vi "RTMain.Write Data.vi"(8 "error in":errorcluster, 9 "WriteUpdate":refnum<k33>, 10 "Read from VS Engine FIFO":refnum<k33>, 11 "Data Refs":T1 {"Write Refs" format="%.0x"; "Read Refs" format="%.0x"}) -> (0 "error out":errorcluster, 3 "Data Refs":T1 {"Write Refs" format="%.0x"; "Read Refs" format="%.0x"})   [LabVIEW 2019, in "OPC UA Client Engine.lvlib"]
uses:
  OPC UA Client Engine.lvlib
  Shared/Tags.ReadWriteRefs.ctl
  <vilib>/NI VeriStand/Custom Device API/Data Reference.ctl
  <vilib>/NI VeriStand/Custom Device API/Global Data Refs.vi
  <vilib>/NI VeriStand/Custom Device API/Custom Device API.lvlib
  Shared/OPC UA Client Shared.lvlib
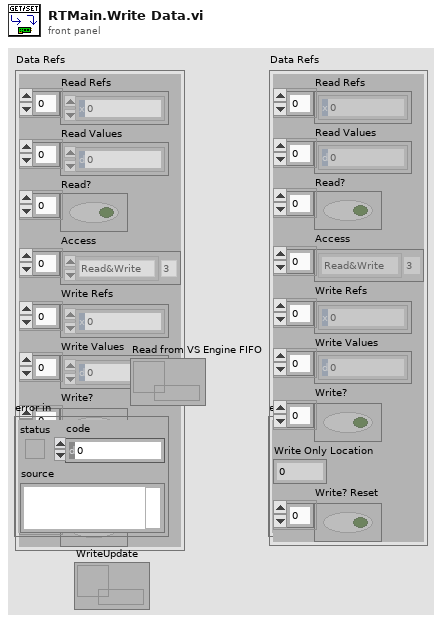
[diagram p1: front panel]
types:
  T1 = typedef "OPC UA Client Shared.lvlib/Tags.ReadWriteRefs.ctl" = cluster{"Read Refs":T2[], "Read Values":dbl[], "Read?":bool[], "Access":enum8{"Null", "Read", "Write", "Read&Write"}[], "Write Refs":T2[], "Write Values":dbl[], "Write?":bool[], "Write Only Location":u32, "Write? Reset":bool[]}
  T2 = typedef "Custom Device API.lvlib/Data Reference.ctl" = i32
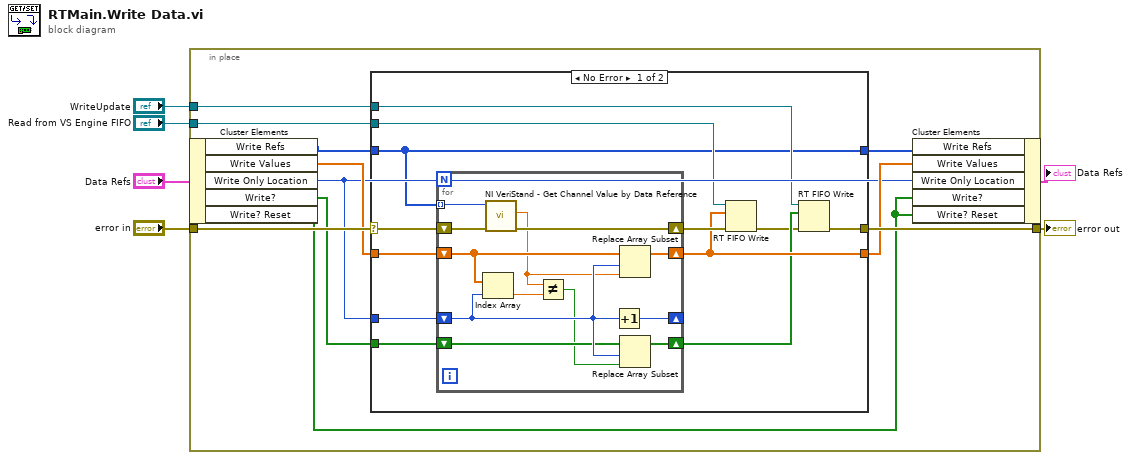
[diagram p0: block diagram]
diagram:
  n1 = in-place {
    in-place-border: [w17] -> w6
    in-place-border: "error in" -> [w16]
    in-place-border: "Read from VS Engine FIFO" -> [w15]
    in-place-border: "WriteUpdate" -> [w11]
    n2 = in-place-cluster #1("Data Refs") -> ("Write Refs"=w10:T2[], "Write Values"=w14:dbl[], "Write Only Location"=w8:u32, "Write?"=w12:bool[], "Write? Reset"=w7:bool[])
    n3 = case shown="No Error" w16 {
      selector: w16 -> [w21 w44]
      tunnel: [w18 w44] -> w17
      tunnel: w15 -> [w29 _]
      tunnel: w14 -> [w20 w43]
      tunnel: [w26 w43] -> w13
      tunnel: w12 -> [w22 _]
      tunnel: w11 -> [w28 _]
      tunnel: w10 -> [w24 w42]
      tunnel: [w24 w42] -> w9
      tunnel: w8 -> [w23 _]
      frame No Error {
        n4 = for {
          shift-right: [w41] -> w27
          shift-left: w21 -> [w40]
          tunnel: w24 -> [w39] mode=indexing
          shift-right: [w37] -> _
          shift-left: w23 -> [w36]
          shift-right: [w35] -> w26
          shift-left: w20 -> [w38]
          shift-right: [w33] -> w25
          shift-left: w22 -> [w34]
          n5 = Index Array(array=w38, index=w36) -> (element=w31:dbl)
          n6 = call <vilib>:"NI VeriStand - Get Channel Value by Data Reference.vi"("error in (no error)"=w40, "Data Reference in"=w39) -> ("error out"=w41:errorcluster, "Value"=w32:dbl)  [unwired: 8 in]
          n7 = Not Equal?(x=w32, y=w31) -> (x != y?=w30:bool)
          n8 = Increment(x=w36) -> (x+1=w37:u32)
          n9 = Replace Array Subset(array=w38, new element=w32, index=w36) -> (w35:dbl[])
          n10 = Replace Array Subset(array=w34, new element=w30, index=w36) -> (w33:bool[])
        }
        n11 = RT FIFO Write(0:w29, 1:w26, 3:w27) -> (11:w19:errorcluster)  [unwired: 2 in, 3 out]
        n12 = RT FIFO Write(0:w28, 1:w25, 3:w19) -> (11:w18:errorcluster)  [unwired: 2 in, 3 out]
      }
      frame Error {
      }
    }
    n13 = in-place-cluster #1("Write Refs"=w9, "Write Values"=w13, "Write Only Location"=w8, "Write?"=w7, "Write? Reset"=w7) -> (→"Data Refs":T1)
  }
  "error out" <- w6
